vi "Add Quotes.vi"(8 "error in (no error)":errorcluster, 11 "string":string) -> (0 "error out":errorcluster, 3 "with quotes":string)   [LabVIEW 2017, in "NI_LVConfig.lvlib"]
doc: "Adds quote marks (\") around a string that contains spaces."
uses:
  <vilib>/Utility/config.llb/NI_LVConfig.lvlib
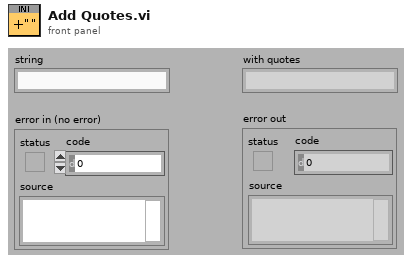
[diagram p1: front panel]
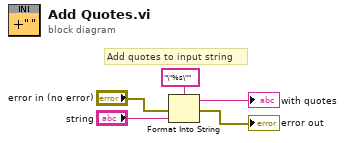
[diagram p0: block diagram]
diagram:
  # "Add quotes to input string"
  n1 = Format Into String(format string="\"%s\"", error in="error in (no error)", "string") -> (resulting string=→"with quotes":string, error out=→"error out":errorcluster)  [unwired: 1 in]
